vi "Update_e_t_ForAmplitudeFeedback.vi"(7 "Rest":bool, 8 "input valid":bool=TRUE, 11 "e(t)":fxp<+/-,33,15>) -> (0 "output valid":bool, 2 "e(t-1)-e(t-2)":fxp<+/-,34,16>, 3 "e(t)-e(t-1)":fxp<+/-,34,16>)   [LabVIEW 2018]
uses:
  <vilib>/rvi/FXPMathLib/FxpSub/XNode/nifxpmath_Sub.xnode
  <vilib>/rvi/FXPMathLib/sim/FxpSim.dll
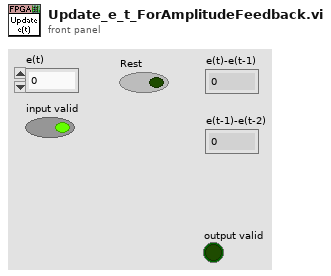
[diagram p1: front panel]
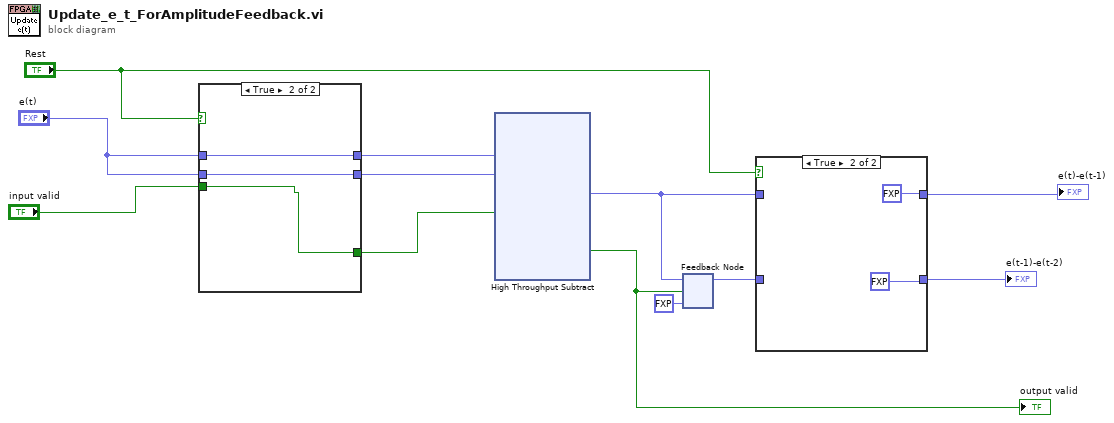
[diagram p0: block diagram]
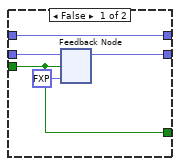
[diagram p3: hidden frame]
diagram:
  n1 = case shown="True" "Rest" {
    tunnel: "e(t)" -> [w17 w19]
    tunnel: [w16 w19] -> w12
    tunnel: "input valid" -> [w14 w18]
    tunnel: "e(t)" -> [w15 w20]
    tunnel: [w15 w20] -> w8
    tunnel: [w14 w18] -> w7
    frame False {
      n2 = feedback #1(fxp<+/-,17,15> 0.0 ("e(t)")) -> (w16:fxp<+/-,33,15>)
      n3 = feedback-in #1(w17, w14) -> ()
    }
    frame True {
    }
  }
  n4 = xnode "High Throughput Subtract"("x"=w8, "y"=w12, "input valid"=w7) -> ("x-y"=w5:fxp<+/-,34,16>, "output valid"=w11:bool)  [unwired: 1 in, 1 out]
  "output valid" <- w11
  n5 = feedback #2(fxp<+/-,34,16> 0.0 ("x-y")) -> (w4:fxp<+/-,34,16>)
  n6 = feedback-in #2(w5, w11) -> ()
  n7 = case shown="True" "Rest" {
    tunnel: w5 -> [w22 _]
    tunnel: w4 -> [w21 _]
    tunnel: [w22 fxp<+/-,34,16> 0.0 ("x-y")] -> w3
    tunnel: [w21 fxp<+/-,34,16> 0.0 ("x-y")] -> w2
    frame False {
    }
    frame True {
    }
  }
  "e(t)-e(t-1)" <- w3
  "e(t-1)-e(t-2)" <- w2
